vi "Read Circle Progress.vi"   [LabVIEW 2011, in "LVH-Leap.lvlib"]
doc: "Read circle gesture progress. Use the polymorphic instance to select between one circle and N circles."
uses:
  LVH-Leap.lvlib
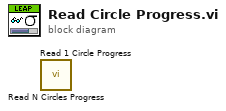
[diagram p0: block diagram]
diagram:
  n1 = call "Read N Circles Progress.vi"() -> ()  [unwired: 9 in, 3 out]
  n2 = call "Read 1 Circle Progress.vi"() -> ()  [unwired: 8 in, 4 out]
